vi "Plot It.vi"(1 "X-Axis":i32(ring)=1 items=["Point #", "Field", "Voltage1"], 2 "Display?":bool[](array[boolean])=[FALSE, FALSE, FALSE, FALSE, FALSE, FALSE, FALSE, FALSE, FALSE, FALSE, FALSE, FALSE, FALSE, FALSE, FALSE, FALSE, FALSE], 3 "# of columns":i32=-10, 4 "Index":i32=-2000000000) -> (0 "?":bool=TRUE)   [LabVIEW 2019]
doc: "This VI decides if there is more data or if the plot parameters have changed. If not then returns false."
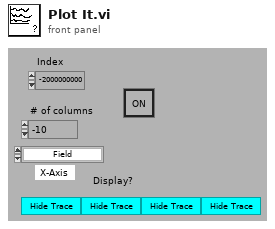
[diagram p1: front panel]
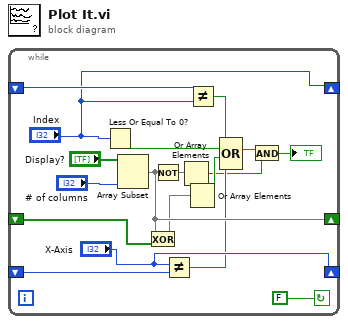
[diagram p0: block diagram]
diagram:
  n1 = while {
    shift-left: _ -> [w8]
    shift-right: ["X-Axis"] -> _
    shift-left: _ -> [w10]
    shift-right: [w11] -> _
    shift-left: _ -> [w14]
    shift-right: ["Index"] -> _
    stop <- FALSE continue-if-true
    n2 = Less Or Equal To 0?(x="Index") -> (x <= 0?=w15:bool)
    n3 = Array Subset(array="Display?", length="# of columns") -> (w11:bool[])  [unwired: 1 in]
    n4 = Exclusive Or(1:w10, 2:w11) -> (0:w9:bool[])
    n5 = Not(x=w11) -> (.not. x?=w2:bool[])
    n6 = Not Equal?(x="X-Axis", y=w8) -> (x != y?=w6:bool)
    n7 = Or Array Elements(Boolean array=w2) -> (logical OR=w3:bool)
    n8 = Or Array Elements(Boolean array=w9) -> (logical OR=w12:bool)
    n9 = Not Equal?(x=w14, y="Index") -> (x != y?=w16:bool)
    n10 = Compound Arithmetic op=OR(w16, w15, w12, w6) -> (w4:bool)
    n11 = And(x=w4, y=w3) -> (x .and. y?=→"?":bool)
  }
